vi "1D Scale n-Exp Parameters.vi"(8 "Error In":errorcluster, 9 "||F||":dbl, 10 "Guess Parameters in":dbl[](array[numeric]), 11 "Fit Model":T1) -> (0 "Error Out":errorcluster, 3 "Guess Parameters out":dbl[](array[numeric]))   [LabVIEW 2021, in "Fits.lvlib"]
uses:
  Decay Convolution/Decay Model.ctl
  <vilib>/Utility/error.llb/Error Cluster From Error Code.vi
  <vilib>/ErrorRing/Error Ring.xnode
  Fits.lvlib
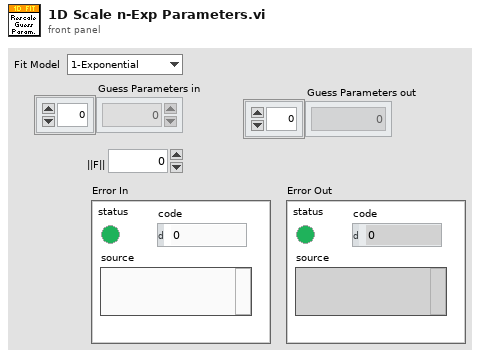
[diagram p1: front panel]
types:
  T1 = typedef "Fits.lvlib/Decay Model.ctl" = enum16{"1-Exponential", "2-Exponentials"}
  T2 = typedef "Fits.lvlib/Decay Fit Parameters In List.ctl" = enum16{"Offset", "Baseline", "A_1", "tau_1", "A_2", "tau_2"}
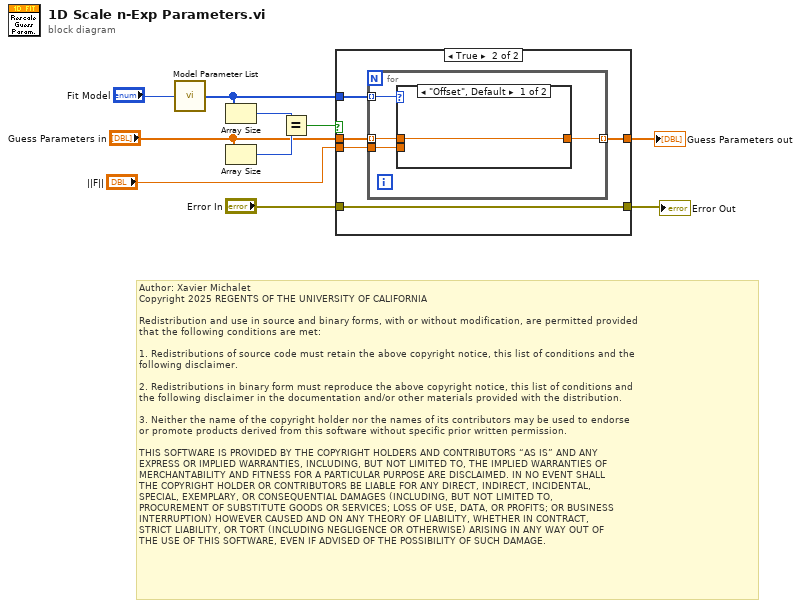
[diagram p0: block diagram]
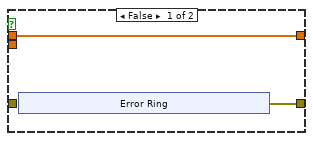
[diagram p2: hidden frame]
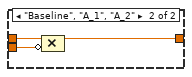
[diagram p3: hidden frame]
diagram:
  # "Author: Xavier Michalet\nCopyright 2025 REGENTS OF THE UNIVERSITY OF CALIFORNIA\n\nRedistribution and use in source and binary forms, with or without modification, are permitted provided\nthat the following conditions are met:\n\n1. Redistributions of source code must retain the above copyright notice, this list of conditions and the\nfollowing disclaimer.\n\n2. Redistributions in binary form must reproduce the above copyright notice, this list of conditions and\nthe following disclaimer in the documentation and/or other materials provided with the distribution.\n\n3. Neither the name of the copyright holder nor the names of its contributors may be used to endorse \nor promote products derived from this software without specific prior written permission.\n\nTHIS SOFTWARE IS PROVIDED BY THE COPYRIGHT HOLDERS AND CONTRIBUTORS “AS IS” AND ANY \nEXPRESS OR IMPLIED WARRANTIES, INCLUDING, BUT NOT LIMITED TO, THE IMPLIED WARRANTIES OF\nMERCHANTABILITY AND FITNESS FOR A PARTICULAR PURPOSE ARE DISCLAIMED. IN NO EVENT SHALL\nTHE COPYRIGHT HOLDER OR CONTRIBUTORS BE LIABLE FOR ANY DIRECT, INDIRECT, INCIDENTAL, \nSPECIAL, EXEMPLARY, OR CONSEQUENTIAL DAMAGES (INCLUDING, BUT NOT LIMITED TO, \nPROCUREMENT OF SUBSTITUTE GOODS OR SERVICES; LOSS OF USE, DATA, OR PROFITS; OR BUSINESS\nINTERRUPTION) HOWEVER CAUSED AND ON ANY THEORY OF LIABILITY, WHETHER IN CONTRACT, \nSTRICT LIABILITY, OR TORT (INCLUDING NEGLIGENCE OR OTHERWISE) ARISING IN ANY WAY OUT OF\nTHE USE OF THIS SOFTWARE, EVEN IF ADVISED OF THE POSSIBILITY OF SUCH DAMAGE."
  n1 = call "Model Parameter List.vi"("Fit Model"="Fit Model") -> ("Model Parameter List"=w4:T2[])
  n2 = Array Size(array=w4) -> (size(s)=w9:i32)
  n3 = Array Size(array="Guess Parameters in") -> (size(s)=w8:i32)
  n4 = Equal?(x=w9, y=w8) -> (x = y?=w7:bool)
  n5 = case shown="True" w7 {
    tunnel: "Guess Parameters in" -> [w12 w19]
    tunnel: [w12 w17] -> w5
    tunnel: w4 -> [_ w20]
    tunnel: [w11 w21] -> w3
    tunnel: "Error In" -> [_ w21]
    tunnel: "||F||" -> [_ w18]
    frame False {
      n6 = xnode "Error Ring"() -> ("error out"=w11:errorcluster)
    }
    frame True {
      n7 = for {
        tunnel: w20 -> [w25] mode=indexing
        tunnel: w19 -> [w24] mode=indexing
        tunnel: w18 -> [w23]
        tunnel: [w22] -> w17 mode=indexing
        n8 = case shown="\"Offset\", Default" w25 {
          tunnel: [w26 w29] -> w22
          tunnel: w24 -> [w26 w28]
          tunnel: w23 -> [_ w27]
          frame "Offset", Default {
          }
          frame "Baseline", "A_1", "A_2" {
            n9 = Compound Arithmetic op=MULTIPLY(w28, invert w27) -> (w29:dbl)
          }
        }
      }
    }
  }
  "Guess Parameters out" <- w5
  "Error Out" <- w3
